vi "Variant.SetName.vi"(9 "Name":string, 10 "Variant":variant) -> (2 "Named Variant":variant)   [LabVIEW 2021, in "json.facade.lvlib"]
uses:
  json.facade.lvlib
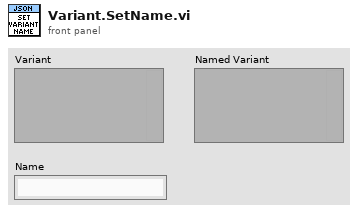
[diagram p1: front panel]
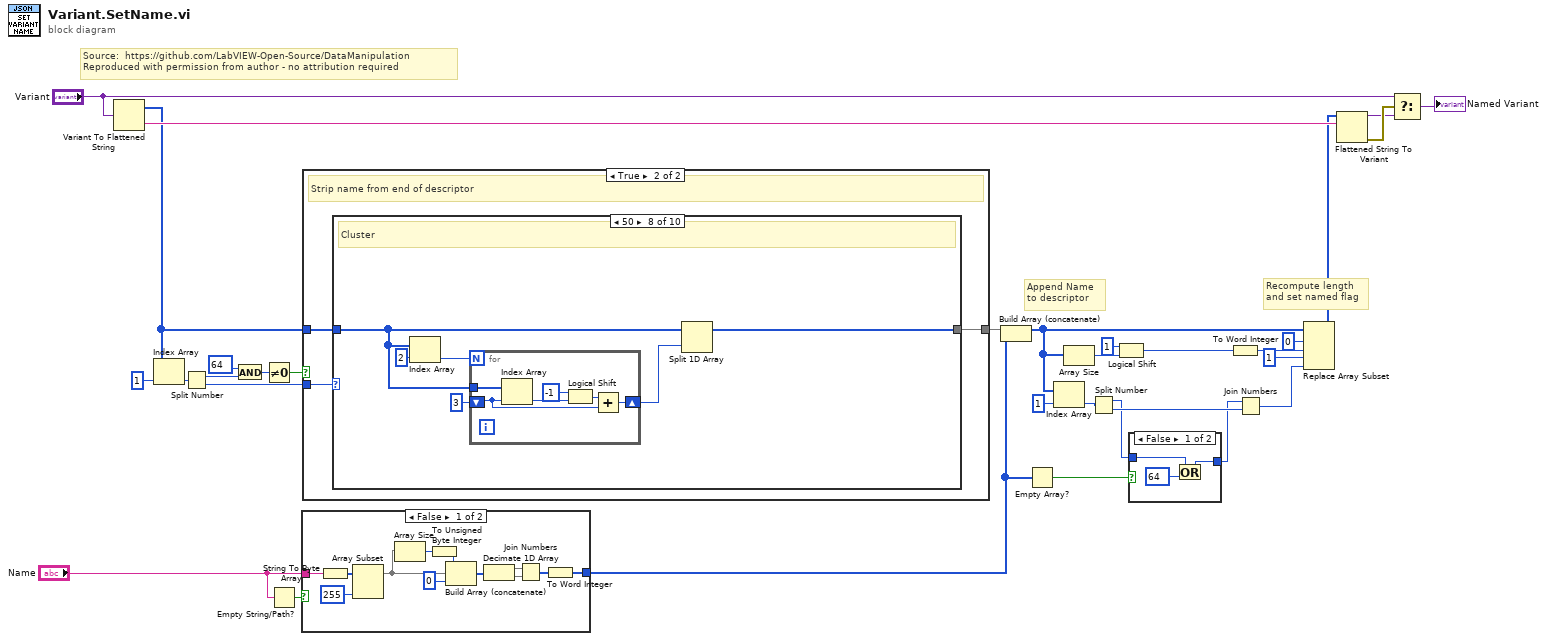
[diagram p0: block diagram]
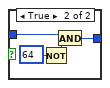
[diagram p2: hidden frame]
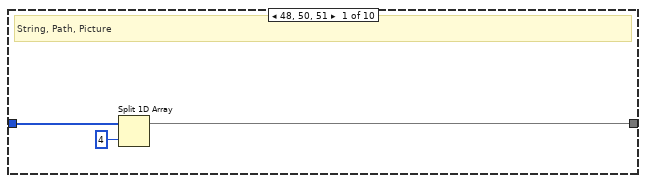
[diagram p5: hidden frame]
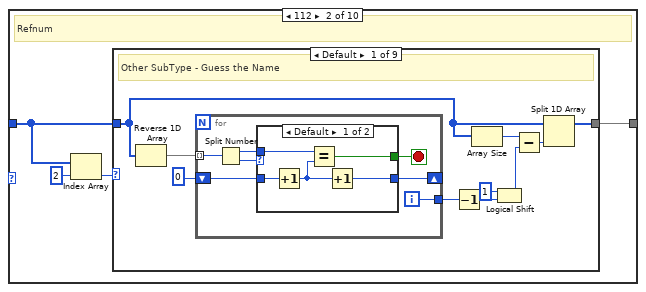
[diagram p6: hidden frame]
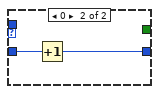
[diagram p7: hidden frame]
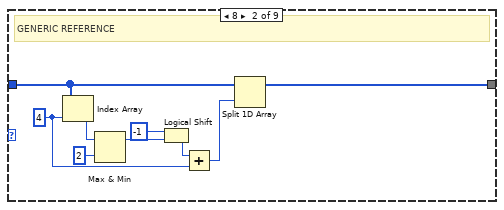
[diagram p8: hidden frame]
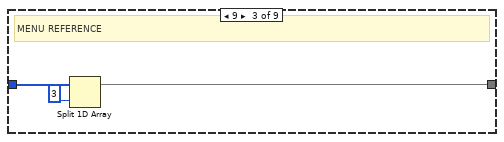
[diagram p9: hidden frame]
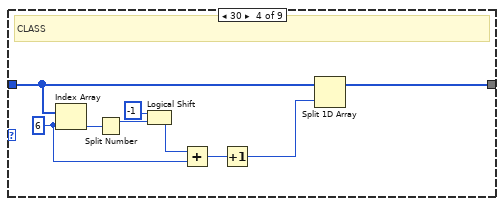
[diagram p10: hidden frame]
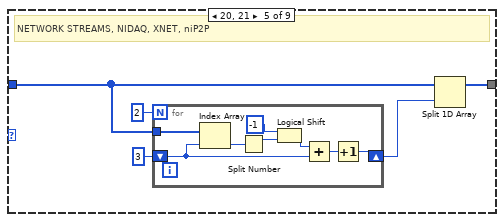
[diagram p11: hidden frame]
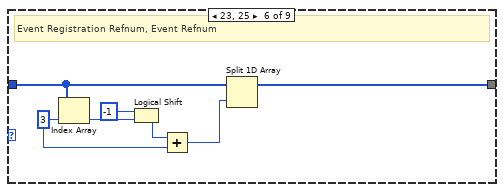
[diagram p12: hidden frame]
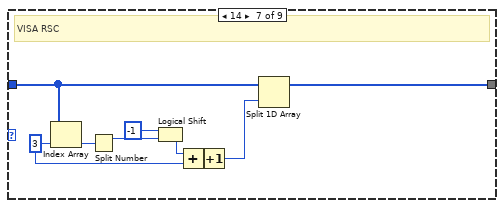
[diagram p13: hidden frame]
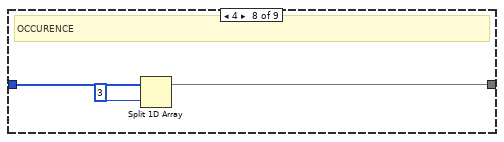
[diagram p14: hidden frame]
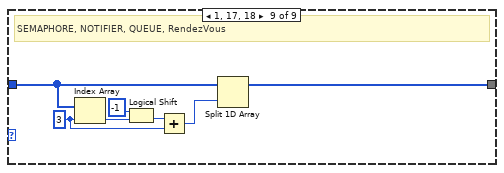
[diagram p15: hidden frame]
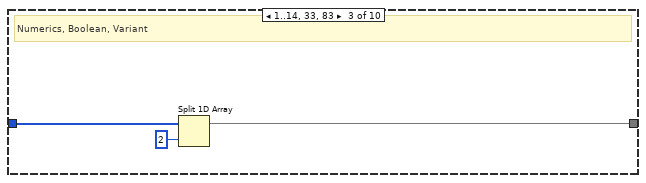
[diagram p16: hidden frame]
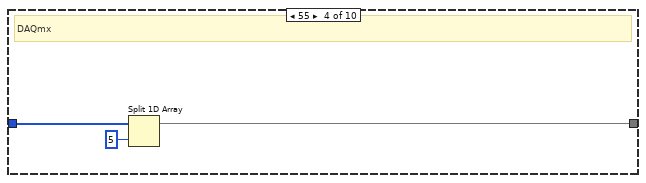
[diagram p17: hidden frame]
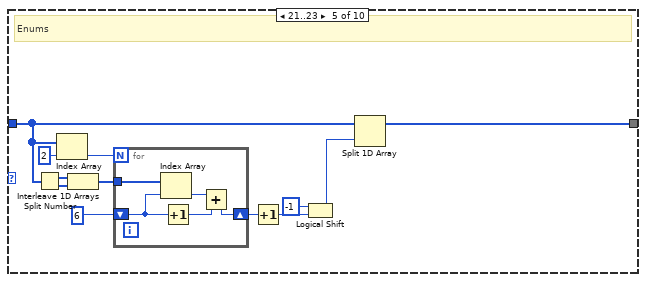
[diagram p18: hidden frame]
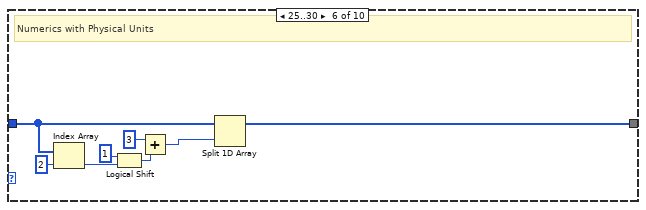
[diagram p19: hidden frame]
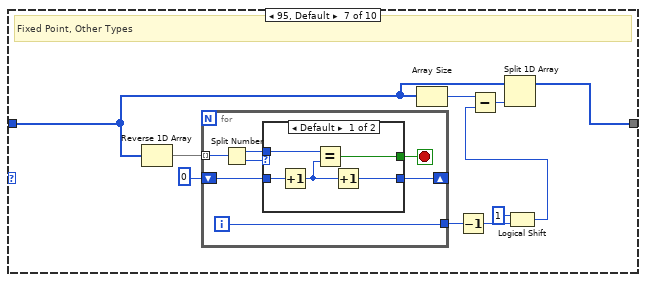
[diagram p20: hidden frame]
diagram:
  # "Source:  https://github.com/LabVIEW-Open-Source/DataManipulation\nReproduced with permission from author - no attribution required"
  # "Recompute length\nand set named flag"
  # "Append Name\nto descriptor"
  n1 = Variant To Flattened String(Variant="Variant") -> (data string=w32:string, 1:w3:i16[])
  n2 = Index Array(array=w3, index=1) -> (element=w27:i16)
  n3 = Split Number(x=w27) -> (hi(x)=w22:u8, lo(x)=w24:u8)
  n4 = And(x=u8 64, y=w22) -> (x .and. y?=w21:u8)
  n5 = Not Equal To 0?(x=w21) -> (x != 0?=w25:bool)
  n6 = Empty String/Path?(string/path="Name") -> (empty?=w20:bool)
  n7 = case shown="False" w20 {
    tunnel: [w34 _] -> w7
    tunnel: "Name" -> [w33 _]
    frame False {
      n8 = String To Byte Array(string=w33) -> (unsigned byte array=w39:u8[])
      n9 = Array Subset(array=w39, length=255) -> (w38:u8[])  [unwired: 1 in]
      n10 = Array Size(array=w38) -> (size(s)=w37:i32)
      n11 = To Unsigned Byte Integer(number=w37) -> (unsigned 8bit integer=w36:u8)
      n12 = Build Array (concatenate)(w36, w38, u8 0) -> (w43:u8[])
      n13 = Decimate 1D Array(w43) -> (w42:u8[], w41:u8[])
      n14 = Join Numbers(hi=w42, lo=w41) -> ((hi.lo)=w35:u16[])
      n15 = To Word Integer(number=w35) -> (16bit integer=w34:i16[])
    }
    frame True {
    }
  }
  n16 = case shown="True" w25 {
    tunnel: w24 -> [_ w47]
    tunnel: [w45 w46] -> w8
    tunnel: w3 -> [w45 w48]
    frame False {
    }
    frame True {
      # "Strip name from end of descriptor"
      n17 = case shown="50" w47 {
        tunnel: w48 -> [w51 w53 w141 w144 w148 w165 w175 w196 w208 w216]
        tunnel: [w49 w52 w140 w143 w146 w163 w176 w195 w209 w215] -> w46
        frame 48, 50, 51 {
          # "String, Path, Picture"
          n18 = Split 1D Array(array=w51, index=4) -> (first subarray=w49:i16[])  [unwired: 1 out]
        }
        frame 112 {
          # "Refnum"
          n19 = Index Array(array=w53, index=2) -> (element=w54:i16)
          n20 = case shown="Default" w54 {
            tunnel: w53 -> [w61 w82 w91 w93 w103 w116 w122 w132 w134]
            tunnel: [w60 w80 w89 w92 w102 w114 w123 w130 w133] -> w52
            frame Default {
              # "Other SubType - Guess the Name"
              n21 = Reverse 1D Array(array=w61) -> (reversed array=w64:i16[])
              n22 = for {
                tunnel: w64 -> [w67] mode=indexing
                shift-right: [w69] -> _
                shift-left: u8 0 ("hi(x)") -> [w70]
                tunnel: [w66] -> w56
                i -> [w66]
                stop <- w68 stop-if-true
                n23 = Split Number(x=w67) -> (hi(x)=w71:u8, lo(x)=w72:u8)
                n24 = case shown="Default" w72 {
                  tunnel: [w73 _] -> w68
                  tunnel: w71 -> [w77 _]
                  tunnel: w70 -> [w76 w79]
                  tunnel: [w74 w78] -> w69
                  frame Default {
                    n25 = Increment(x=w76) -> (x+1=w75:u8)
                    n26 = Equal?(x=w77, y=w75) -> (x = y?=w73:bool)
                    n27 = Increment(x=w75) -> (x+1=w74:u8)
                  }
                  frame 0 {
                    n28 = Increment(x=w79) -> (x+1=w78:u8)
                  }
                }
              }
              n29 = Decrement(x=w56) -> (x-1=w58:i32)
              n30 = Array Size(array=w61) -> (size(s)=w63:i32)
              n31 = Logical Shift(y=i16 1, x=w58) -> (x << y=w57:i32)
              n32 = Subtract(x=w63, y=w57) -> (x-y=w62:i32)
              n33 = Split 1D Array(array=w61, index=w62) -> (first subarray=w60:i16[])  [unwired: 1 out]
            }
            frame 8 {
              w86 = 4 ("index")
              # "GENERIC REFERENCE"
              n34 = Index Array(array=w82, index=w86) -> (element=w84:i16)
              n35 = Max & Min(x=w84, y=i16 2) -> (max(x,y)=w85:i16)  [unwired: 1 out]
              n36 = Logical Shift(y=i16 -1, x=w85) -> (x << y=w87:i16)
              n37 = Add(x=w87, y=w86) -> (x+y=w81:i32)
              n38 = Split 1D Array(array=w82, index=w81) -> (first subarray=w80:i16[])  [unwired: 1 out]
            }
            frame 9 {
              # "MENU REFERENCE"
              n39 = Split 1D Array(array=w91, index=3) -> (first subarray=w89:i16[])  [unwired: 1 out]
            }
            frame 30 {
              w96 = 6 ("index")
              # "CLASS"
              n40 = Index Array(array=w93, index=w96) -> (element=w100:i16)
              n41 = Split Number(x=w100) -> (hi(x)=w99:u8)  [unwired: 1 out]
              n42 = Logical Shift(y=i16 -1, x=w99) -> (x << y=w97:u8)
              n43 = Add(x=w97, y=w96) -> (x+y=w95:i32)
              n44 = Increment(x=w95) -> (x+1=w94:i32)
              n45 = Split 1D Array(array=w93, index=w94) -> (first subarray=w92:i16[])  [unwired: 1 out]
            }
            frame 20, 21 {
              # "NETWORK STREAMS, NIDAQ, XNET, niP2P"
              n46 = for {
                N: 2 -> [_]
                shift-right: [w112] -> w101
                shift-left: 3 ("index") -> [w110]
                tunnel: w103 -> [w111]
                n47 = Index Array(array=w111, index=w110) -> (element=w107:i16)
                n48 = Split Number(x=w107) -> (hi(x)=w109:u8)  [unwired: 1 out]
                n49 = Logical Shift(y=i16 -1, x=w109) -> (x << y=w106:u8)
                n50 = Add(x=w106, y=w110) -> (x+y=w113:i32)
                n51 = Increment(x=w113) -> (x+1=w112:i32)
              }
              n52 = Split 1D Array(array=w103, index=w101) -> (first subarray=w102:i16[])  [unwired: 1 out]
            }
            frame 23, 25 {
              w118 = 3 ("index")
              # "Event Registration Refnum, Event Refnum"
              n53 = Index Array(array=w116, index=w118) -> (element=w117:i16)
              n54 = Logical Shift(y=i16 -1, x=w117) -> (x << y=w119:i16)
              n55 = Add(x=w119, y=w118) -> (x+y=w115:i32)
              n56 = Split 1D Array(array=w116, index=w115) -> (first subarray=w114:i16[])  [unwired: 1 out]
            }
            frame 14 {
              w127 = 3 ("index")
              # "VISA RSC"
              n57 = Index Array(array=w122, index=w127) -> (element=w125:i16)
              n58 = Split Number(x=w125) -> (hi(x)=w124:u8)  [unwired: 1 out]
              n59 = Logical Shift(y=i16 -1, x=w124) -> (x << y=w128:u8)
              n60 = Add(x=w128, y=w127) -> (x+y=w126:i32)
              n61 = Increment(x=w126) -> (x+1=w121:i32)
              n62 = Split 1D Array(array=w122, index=w121) -> (first subarray=w123:i16[])  [unwired: 1 out]
            }
            frame 4 {
              # "OCCURENCE"
              n63 = Split 1D Array(array=w132, index=3 ("offset (0)")) -> (first subarray=w130:i16[])  [unwired: 1 out]
            }
            frame 1, 17, 18 {
              w137 = 3 ("index")
              # "SEMAPHORE, NOTIFIER, QUEUE, RendezVous"
              n64 = Index Array(array=w134, index=w137) -> (element=w139:i16)
              n65 = Logical Shift(y=i16 -1, x=w139) -> (x << y=w136:i16)
              n66 = Add(x=w136, y=w137) -> (x+y=w135:i32)
              n67 = Split 1D Array(array=w134, index=w135) -> (first subarray=w133:i16[])  [unwired: 1 out]
            }
          }
        }
        frame 1..14, 33, 83 {
          # "Numerics, Boolean, Variant"
          n68 = Split 1D Array(array=w141, index=2) -> (first subarray=w140:i16[])  [unwired: 1 out]
        }
        frame 55 {
          # "DAQmx"
          n69 = Split 1D Array(array=w144, index=5) -> (first subarray=w143:i16[])  [unwired: 1 out]
        }
        frame 21..23 {
          # "Enums"
          n70 = Split Number(x=w148) -> (hi(x)=w152:u8[], lo(x)=w151:u8[])
          n71 = Index Array(array=w148, index=2) -> (element=w156:i16)
          n72 = Interleave 1D Arrays(w152, w151) -> (w150:u8[])
          n73 = for {
            N: w156 -> [_]
            shift-right: [w160] -> w153
            shift-left: 6 ("index") -> [w159]
            tunnel: w150 -> [w162]
            n74 = Index Array(array=w162, index=w159) -> (element=w161:u8)
            n75 = Increment(x=w159) -> (x+1=w158:i32)
            n76 = Add(x=w161, y=w158) -> (x+y=w160:i32)
          }
          n77 = Increment(x=w153) -> (x+1=w149:i32)
          n78 = Logical Shift(y=i16 -1, x=w149) -> (x << y=w147:i32)
          n79 = Split 1D Array(array=w148, index=w147) -> (first subarray=w146:i16[])  [unwired: 1 out]
        }
        frame 25..30 {
          # "Numerics with Physical Units"
          n80 = Index Array(array=w165, index=2) -> (element=w168:i16)
          n81 = Logical Shift(y=i16 1, x=w168) -> (x << y=w167:i16)
          n82 = Add(x=3, y=w167) -> (x+y=w164:i32)
          n83 = Split 1D Array(array=w165, index=w164) -> (first subarray=w163:i16[])  [unwired: 1 out]
        }
        frame 95, Default {
          # "Fixed Point, Other Types"
          n84 = Reverse 1D Array(array=w175) -> (reversed array=w179:i16[])
          n85 = for {
            tunnel: w179 -> [w182] mode=indexing
            shift-right: [w184] -> _
            shift-left: u8 0 ("hi(x)") -> [w185]
            tunnel: [w181] -> w172
            i -> [w181]
            stop <- w183 stop-if-true
            n86 = Split Number(x=w182) -> (hi(x)=w186:u8, lo(x)=w187:u8)
            n87 = case shown="Default" w187 {
              tunnel: [w188 _] -> w183
              tunnel: w186 -> [w192 _]
              tunnel: w185 -> [w191 w194]
              tunnel: [w189 w193] -> w184
              frame Default {
                n88 = Increment(x=w191) -> (x+1=w190:u8)
                n89 = Equal?(x=w192, y=w190) -> (x = y?=w188:bool)
                n90 = Increment(x=w190) -> (x+1=w189:u8)
              }
              frame 0 {
                n91 = Increment(x=w194) -> (x+1=w193:u8)
              }
            }
          }
          n92 = Array Size(array=w175) -> (size(s)=w178:i32)
          n93 = Decrement(x=w172) -> (x-1=w171:i32)
          n94 = Logical Shift(y=i16 1, x=w171) -> (x << y=w173:i32)
          n95 = Subtract(x=w178, y=w173) -> (x-y=w177:i32)
          n96 = Split 1D Array(array=w175, index=w177) -> (first subarray=w176:i16[])  [unwired: 1 out]
        }
        frame 80 {
          # "Cluster"
          n97 = Index Array(array=w196, index=2) -> (element=w199:i16)
          n98 = for {
            N: w199 -> [_]
            tunnel: w196 -> [w206]
            shift-right: [w201] -> w197
            shift-left: 3 ("index") -> [w202]
            n99 = Index Array(array=w206, index=w202) -> (element=w204:i16)
            n100 = Logical Shift(y=i16 -1, x=w204) -> (x << y=w203:i16)
            n101 = Add(x=w203, y=w202) -> (x+y=w201:i32)
          }
          n102 = Split 1D Array(array=w196, index=w197) -> (first subarray=w195:i16[])  [unwired: 1 out]
        }
        frame 84 {
          # "Waveforms, Timestamp"
          n103 = Index Array(array=w208, index=3) -> (element=w212:i16)
          n104 = Logical Shift(y=i16 -1, x=w212) -> (x << y=w211:i16)
          n105 = Add(x=3 ("y"), y=w211) -> (x+y=w207:i32)
          n106 = Split 1D Array(array=w208, index=w207) -> (first subarray=w209:i16[])  [unwired: 1 out]
        }
        frame 64 {
          # "Arrays"
          n107 = Index Array(array=w216, index=2) -> (element=w221:i16)
          n108 = Logical Shift(y=i16 1, x=w221) -> (x << y=w220:i16)
          n109 = Add(x=w220, y=3) -> (x+y=w219:i32)
          n110 = Index Array(array=w216, index=w219) -> (element=w222:i16)
          n111 = Logical Shift(y=i16 -1, x=w222) -> (x << y=w218:i16)
          n112 = Add(x=w218, y=w219) -> (x+y=w217:i32)
          n113 = Split 1D Array(array=w216, index=w217) -> (first subarray=w215:i16[])  [unwired: 1 out]
        }
      }
    }
  }
  n114 = Build Array (concatenate)(w8, w7) -> (w15:i16[])
  n115 = Empty Array?(array=w7) -> (empty?=w6:bool)
  n116 = Index Array(array=w15, index=1) -> (element=w16:i16)
  n117 = Array Size(array=w15) -> (size(s)=w9:i32)
  n118 = Split Number(x=w16) -> (hi(x)=w5:u8, lo(x)=w17:u8)
  n119 = Logical Shift(y=i16 1, x=w9) -> (x << y=w12:i32)
  n120 = case shown="False" w6 {
    tunnel: w5 -> [w228 w231]
    tunnel: [w229 w230] -> w4
    frame False {
      n121 = Or(x=w228, y=u8 64 ("x")) -> (x .or. y?=w229:u8)
    }
    frame True {
      n122 = Not(x=u8 64) -> (.not. x?=w233:u8)
      n123 = And(x=w231, y=w233) -> (x .and. y?=w230:u8)
    }
  }
  n124 = To Word Integer(number=w12) -> (16bit integer=w13:i16)
  n125 = Join Numbers(hi=w4, lo=w17) -> ((hi.lo)=w19:u16)
  n126 = Replace Array Subset(array=w15, new element #1=w13, index #1=0 ("index"), new element #2=w19, index #2=1 ("index")) -> (w1:i16[])
  n127 = Flattened String To Variant(6:w32, 7:w1) -> (0:w31:errorcluster, 3:w30:variant)  [unwired: 1 in]
  n128 = Select(t="Variant", s=w31, f=w30) -> (s? t:f=→"Named Variant":variant)
